vi "FPGA_PPG_check_file_syntax.vi"(1 "cmd_data":string[](array[string]), 4 "cmd":string, 9 "jump_data_tmp_in":u32[](array[numeric])) -> (11 "jump_data_tmp_out":u32[](array[numeric]), 16 "cmd_line":string, 18 "codeOfError":i32)   [LabVIEW 2014, in "NI-FPGA_PPG_Driver.lvlib"]
doc: "Checks the syntax of a command data read from a file and converts the data to a cmd_line that is understood by higher level VIs."
uses:
  NI-FPGA_PPG_Driver.lvlib
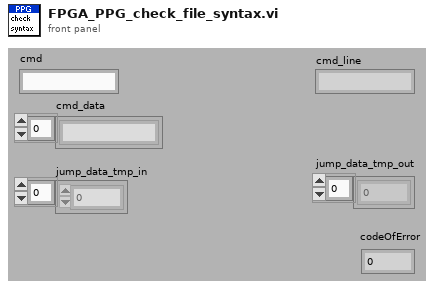
[diagram p1: front panel]
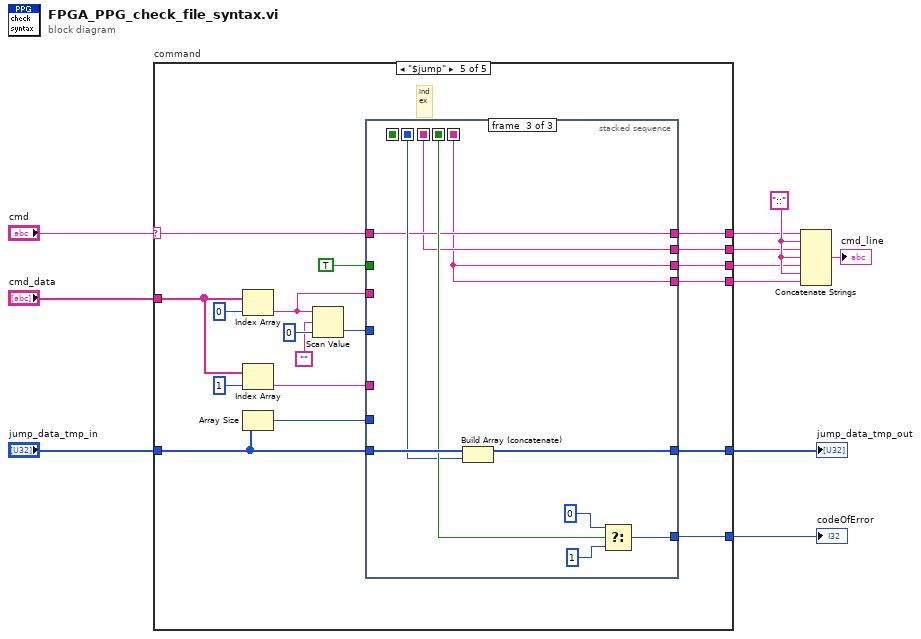
[diagram p0: block diagram]
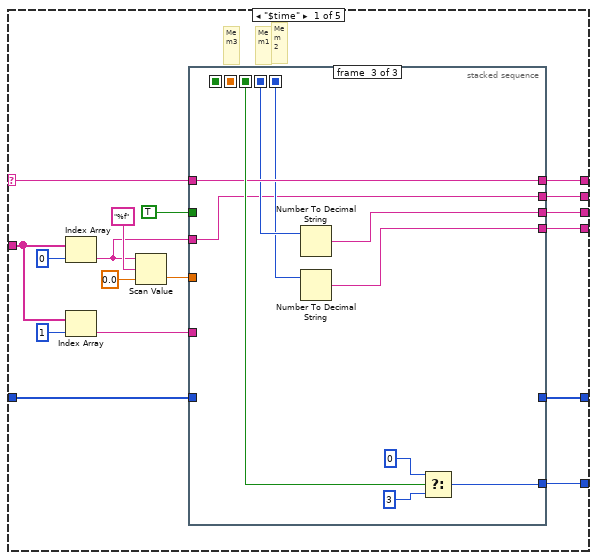
[diagram p2: hidden frame]
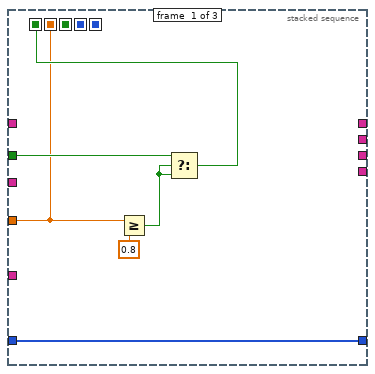
[diagram p3: hidden frame]
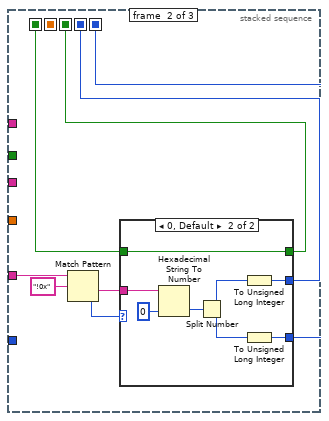
[diagram p4: hidden frame]
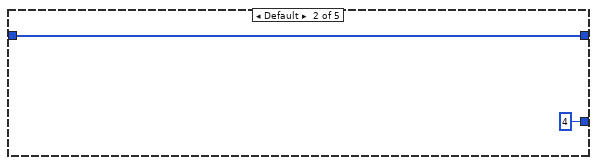
[diagram p6: hidden frame]
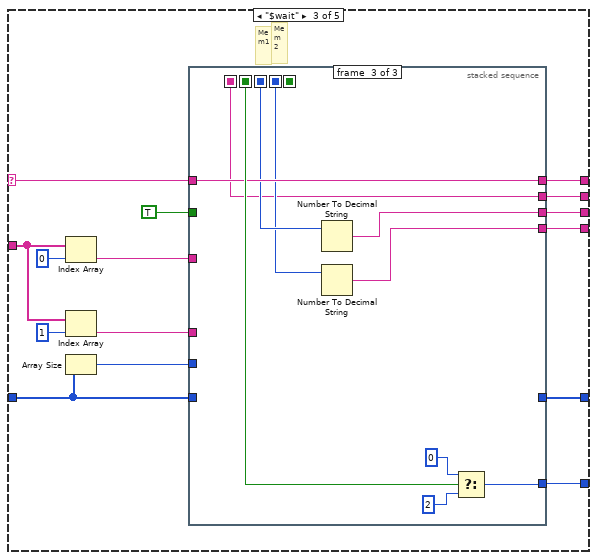
[diagram p7: hidden frame]
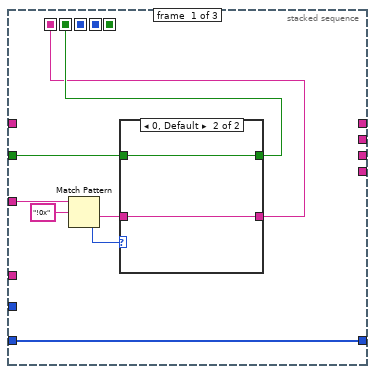
[diagram p8: hidden frame]
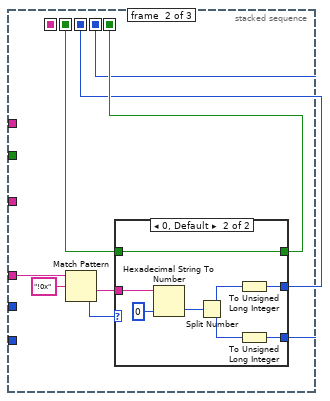
[diagram p10: hidden frame]
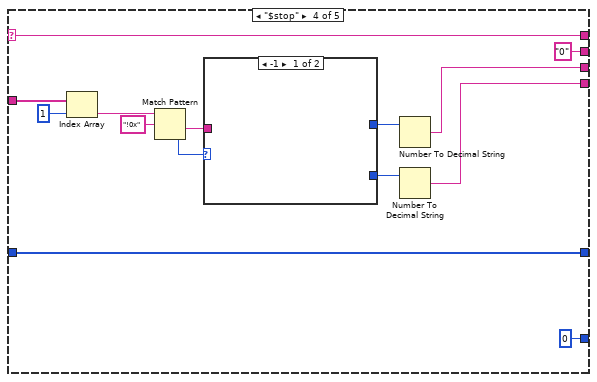
[diagram p12: hidden frame]
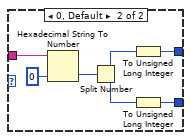
[diagram p13: hidden frame]
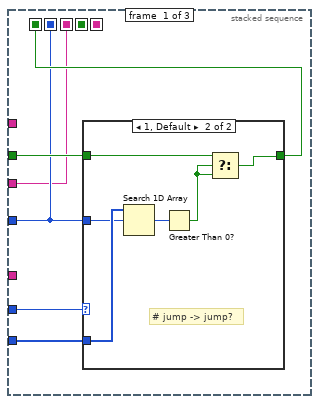
[diagram p14: hidden frame]
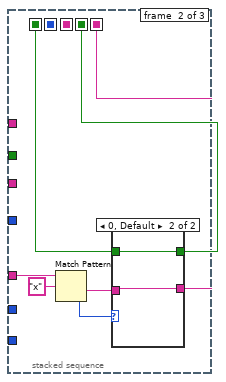
[diagram p16: hidden frame]
diagram:
  w6 = "::"
  n1 = case "command" shown="\"$jump\"" "cmd" {
    selector: "cmd" -> [w17 _ w67 w119 w148]
    tunnel: "jump_data_tmp_in" -> [w19 w62 w70 w127 w150]
    tunnel: "cmd_data" -> [w26 _ w75 w121 w152]
    tunnel: [w20 4 ("f") w71 0 ("f") w151] -> w8
    tunnel: [w18 w62 w68 w127 w149] -> w7
    tunnel: [w16 _ w66 w119 w147] -> w5
    tunnel: [w15 _ w65 "0" ("String") w146] -> w4
    tunnel: [w14 _ w64 w115 w145] -> w3
    tunnel: [w13 _ w63 w114 w144] -> w2
    frame "$time" {
      # "Mem 2"
      # "Mem1"
      # "Mem3"
      n2 = Index Array(array=w26, index=0) -> (element=w12:string)
      n3 = Index Array(array=w26, index=1) -> (element=w21:string)
      n4 = Scan Value(string=w12, format string="%f", default (0 dbl)=0.0) -> (value=w23:dbl)  [unwired: 1 out]
      n5 = stacked-sequence {
        seq-local: [w32 _ _] -> [_ w38 _]
        seq-local: [w29 _ _] -> [_ _ _]
        seq-local: [_ w37 _] -> [_ _ w55]
        seq-local: [_ w36 _] -> [_ _ w53]
        seq-local: [_ w35 _] -> [_ _ w60]
        tunnel: w23 -> [w29 _ _]
        tunnel: TRUE -> [w34 _ _]
        tunnel: w21 -> [_ w42 _]
        tunnel: [_ _ w58] -> w20
        tunnel: w19 -> [w31 _ _]
        tunnel: [w31 _ _] -> w18
        tunnel: w17 -> [_ _ w56]
        tunnel: [_ _ w56] -> w16
        tunnel: [_ _ w51] -> w15
        tunnel: [_ _ w54] -> w14
        tunnel: [_ _ w52] -> w13
        tunnel: w12 -> [_ _ w51]
        frame #0 {
          n6 = Greater Or Equal?(x=w29, y=0.8) -> (x >= y?=w33:bool)
          n7 = Select(t=w34, s=w33, f=w33) -> (s? t:f=w32:bool)
        }
        frame #1 {
          n8 = Match Pattern(string=w42, regular expression="!0x") -> (after substring=w39:string, offset past match=w40:i32)  [unwired: 1 in, 2 out]
          n9 = case shown="0, Default" w40 {
            tunnel: w39 -> [_ w50]
            tunnel: w38 -> [_ w43]
            tunnel: [_ w45] -> w37
            tunnel: [_ w44] -> w36
            tunnel: [_ w43] -> w35
            frame -1 {
            }
            frame 0, Default {
              n10 = Hexadecimal String To Number(string=w50, default (0uL)=u64 0 ("default (0 U32)")) -> (number=w48:u64)  [unwired: 1 in, 1 out]
              n11 = Split Number(x=w48) -> (hi(x)=w47:u32, lo(x)=w46:u32)
              n12 = To Unsigned Long Integer(number=w47) -> (unsigned 32bit integer=w45:u32)
              n13 = To Unsigned Long Integer(number=w46) -> (unsigned 32bit integer=w44:u32)
            }
          }
        }
        frame #2 {
          n14 = Number To Decimal String(number=w55) -> (decimal integer string=w54:string)  [unwired: 1 in]
          n15 = Number To Decimal String(number=w53) -> (decimal integer string=w52:string)  [unwired: 1 in]
          n16 = Select(t=0, s=w60, f=3) -> (s? t:f=w58:i32)
        }
      }
    }
    frame Default {
    }
    frame "$wait" {
      # "Mem 2"
      # "Mem1"
      n17 = Index Array(array=w75, index=0) -> (element=w69:string)
      n18 = Index Array(array=w75, index=1) -> (element=w72:string)
      n19 = Array Size(array=w70) -> (size(s)=w73:i32)
      n20 = stacked-sequence {
        seq-local: [w78 _ _] -> [_ _ w106]
        seq-local: [_ w89 _] -> [_ _ w108]
        seq-local: [_ w88 _] -> [_ _ w107]
        seq-local: [w82 _ _] -> [_ w91 w113]
        seq-local: [_ w90 _] -> [_ _ _]
        tunnel: TRUE -> [w81 _ _]
        tunnel: w73 -> [_ _ _]
        tunnel: w72 -> [_ w92 _]
        tunnel: [_ _ w111] -> w71
        tunnel: w70 -> [w79 _ _]
        tunnel: w69 -> [w80 _ _]
        tunnel: [w79 _ _] -> w68
        tunnel: w67 -> [_ _ w109]
        tunnel: [_ _ w109] -> w66
        tunnel: [_ _ w106] -> w65
        tunnel: [_ _ w105] -> w64
        tunnel: [_ _ w104] -> w63
        frame #0 {
          n21 = Match Pattern(string=w80, regular expression="!0x") -> (after substring=w83:string, offset past match=w84:i32)  [unwired: 1 in, 2 out]
          n22 = case shown="0, Default" w84 {
            tunnel: w83 -> [_ w86]
            tunnel: w81 -> [_ w87]
            tunnel: [_ w87] -> w82
            tunnel: [_ w86] -> w78
            frame -1 {
            }
            frame 0, Default {
            }
          }
        }
        frame #1 {
          n23 = Match Pattern(string=w92, regular expression="!0x") -> (after substring=w93:string, offset past match=w94:i32)  [unwired: 1 in, 2 out]
          n24 = case shown="0, Default" w94 {
            tunnel: w93 -> [_ w103]
            tunnel: w91 -> [_ w96]
            tunnel: [_ w98] -> w89
            tunnel: [_ w97] -> w88
            tunnel: [_ w96] -> w90
            frame -1 {
            }
            frame 0, Default {
              n25 = Hexadecimal String To Number(string=w103, default (0uL)=u64 0 ("default (0 U32)")) -> (number=w101:u64)  [unwired: 1 in, 1 out]
              n26 = Split Number(x=w101) -> (hi(x)=w100:u32, lo(x)=w99:u32)
              n27 = To Unsigned Long Integer(number=w100) -> (unsigned 32bit integer=w98:u32)
              n28 = To Unsigned Long Integer(number=w99) -> (unsigned 32bit integer=w97:u32)
            }
          }
        }
        frame #2 {
          n29 = Number To Decimal String(number=w108) -> (decimal integer string=w105:string)  [unwired: 1 in]
          n30 = Number To Decimal String(number=w107) -> (decimal integer string=w104:string)  [unwired: 1 in]
          n31 = Select(t=0, s=w113, f=2) -> (s? t:f=w111:i32)
        }
      }
    }
    frame "$stop" {
      n32 = Index Array(array=w121, index=1) -> (element=w120:string)
      n33 = Match Pattern(string=w120, regular expression="!0x") -> (after substring=w123:string, offset past match=w124:i32)  [unwired: 1 in, 2 out]
      n34 = case shown="-1" w124 {
        tunnel: w123 -> [_ w134]
        tunnel: [_ w129] -> w117
        tunnel: [_ w128] -> w116
        frame -1 {
        }
        frame 0, Default {
          n35 = Hexadecimal String To Number(string=w134, default (0uL)=u64 0 ("default (0 U32)")) -> (number=w132:u64)  [unwired: 1 in, 1 out]
          n36 = Split Number(x=w132) -> (hi(x)=w131:u32, lo(x)=w130:u32)
          n37 = To Unsigned Long Integer(number=w131) -> (unsigned 32bit integer=w129:u32)
          n38 = To Unsigned Long Integer(number=w130) -> (unsigned 32bit integer=w128:u32)
        }
      }
      n39 = Number To Decimal String(number=w117) -> (decimal integer string=w115:string)  [unwired: 1 in]
      n40 = Number To Decimal String(number=w116) -> (decimal integer string=w114:string)  [unwired: 1 in]
    }
    frame "$jump" {
      # "index"
      n41 = Index Array(array=w152, index=0) -> (element=w135:string)
      n42 = Index Array(array=w152, index=1) -> (element=w136:string)
      n43 = Array Size(array=w150) -> (size(s)=w137:i32)
      n44 = Scan Value(string=w135, format string="", default (0 dbl)=u32 0) -> (value=w139:u32)  [unwired: 1 out]
      n45 = stacked-sequence {
        seq-local: [w155 _ _] -> [_ w168 _]
        seq-local: [w153 _ _] -> [_ _ w176]
        seq-local: [_ w166 _] -> [_ _ w175]
        seq-local: [_ w167 _] -> [_ _ w182]
        seq-local: [w154 _ _] -> [_ _ w179]
        tunnel: w139 -> [w154 _ _]
        tunnel: TRUE -> [w156 _ _]
        tunnel: w137 -> [w158 _ _]
        tunnel: w136 -> [_ w172 _]
        tunnel: [_ _ w180] -> w151
        tunnel: w150 -> [w157 _ w184]
        tunnel: [_ _ w183] -> w149
        tunnel: w148 -> [_ _ w177]
        tunnel: [_ _ w177] -> w147
        tunnel: [_ _ w176] -> w146
        tunnel: [_ _ w175] -> w145
        tunnel: [_ _ w175] -> w144
        tunnel: w135 -> [w153 _ _]
        frame #0 {
          n46 = case shown="1, Default" w158 {
            tunnel: w154 -> [_ w160]
            tunnel: w157 -> [_ w165]
            tunnel: w156 -> [w159 w163]
            tunnel: [w159 w161] -> w155
            frame 0 {
            }
            frame 1, Default {
              # "# jump -> jump?"
              n47 = Search 1D Array(1D array=w165, element=w160) -> (index of element=w164:i32)  [unwired: 1 in]
              n48 = Greater Than 0?(x=w164) -> (x > 0?=w162:bool)
              n49 = Select(t=w163, s=w162, f=w162) -> (s? t:f=w161:bool)
            }
          }
        }
        frame #1 {
          n50 = Match Pattern(string=w172, regular expression="x") -> (after substring=w169:string, offset past match=w170:i32)  [unwired: 1 in, 2 out]
          n51 = case shown="0, Default" w170 {
            tunnel: w169 -> [_ w173]
            tunnel: w168 -> [_ w174]
            tunnel: [_ w174] -> w167
            tunnel: [_ w173] -> w166
            frame -1 {
            }
            frame 0, Default {
            }
          }
        }
        frame #2 {
          n52 = Build Array (concatenate)(w184, w179) -> (w183:u32[])
          n53 = Select(t=0, s=w182, f=1) -> (s? t:f=w180:i32)
        }
      }
    }
  }
  "codeOfError" <- w8
  "jump_data_tmp_out" <- w7
  n54 = Concatenate Strings(w5, w6, w4, w6, w3, w6, w2) -> (→"cmd_line":string)
